vi "Calculate Joint Accelerations.vi"(0 "serial arm in":refnum<class "NI_Robotics_Serial Robot Arm.lvclass">, 5 "joint positions":dbl[](array[numeric]), 7 "joint velocities":dbl[](array[numeric]), 9 "torques":dbl[](array[numeric]), 11 "error in (no error)":errorcluster) -> (4 "serial arm out":refnum<class "NI_Robotics_Serial Robot Arm.lvclass">, 6 "joint accelerations":dbl[](array[numeric]), 15 "error out":errorcluster)   [LabVIEW 2017, in "NI_Kinematics.lvlib"]
doc: "Calculates the <B>joint accelerations</B> that result from applying <B>torques</B> to a robotic arm.\n\n<B>.m file:</B> accel"
uses:
  <vilib>/robotics/Kinematics/NI_Kinematics.lvlib
  <vilib>/robotics/Kinematics/Robot/NI_Robotics_Serial Robot Arm.lvclass
  <vilib>/Analysis/Matrix/Datatypes/RealMatrix.ctl
  <vilib>/Analysis/baseanly.llb/Real Outer Product.vi
  <vilib>/Analysis/7linalg.llb/Solve Linear Equations (single right hand).vi
  <vilib>/Analysis/baseanly.llb/Solve Linear Equations By Cholesky.vi
  <vilib>/Analysis/baseanly.llb/Real Matrix to Compact Array.vi
  <vilib>/Analysis/baseanly.llb/Real Compact Tri-Matrix Linear Eqs.vi
  <vilib>/Analysis/7linalg.llb/Solve Linear Eqs (General).vi
  <vilib>/Analysis/7linalg.llb/Solve Linear Eqs (Gen, single right hand).vi
  <vilib>/robotics/Kinematics/dyn/Inverse Dynamics (Point).vi
  <vilib>/Analysis/Matrix/Numeric/Conversions/Array To Matrix - RA2.vi
  <vilib>/robotics/Kinematics/dyn/Inverse Dynamics (Trajectory).vi
  <vilib>/Analysis/7linalg.llb/Create Special Real Matrix.vi
  <vilib>/Analysis/NI_AALBase.lvlib
  <vilib>/Analysis/Matrix/NI_Matrix.lvlib
  <vilib>/Analysis/NI_AALPro.lvlib
  <vilib>/robotics/Utilities/NI_Robotics Utilities.lvlib
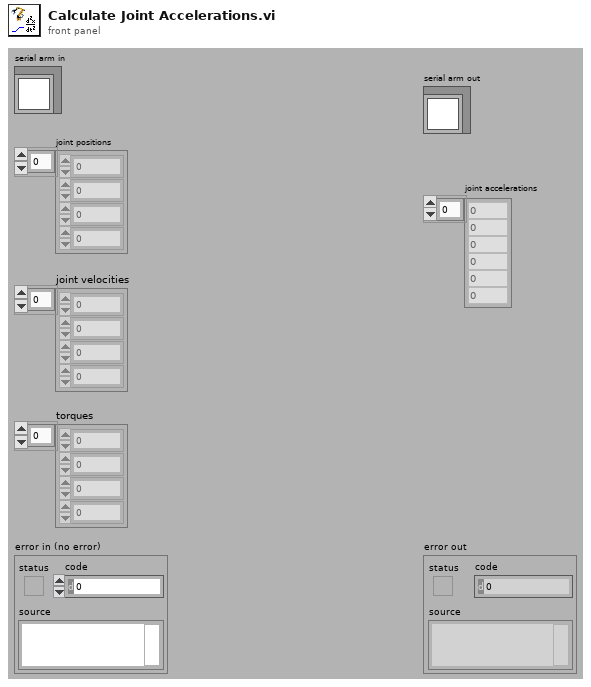
[diagram p1: front panel]
types:
  T1 = enum32{"Identity", "Diagonal", "Toepliz", "Vandermonde", "Companion"}
  T2 = typedef "NI_Matrix.lvlib/RealMatrix.ctl" = dbl[][]
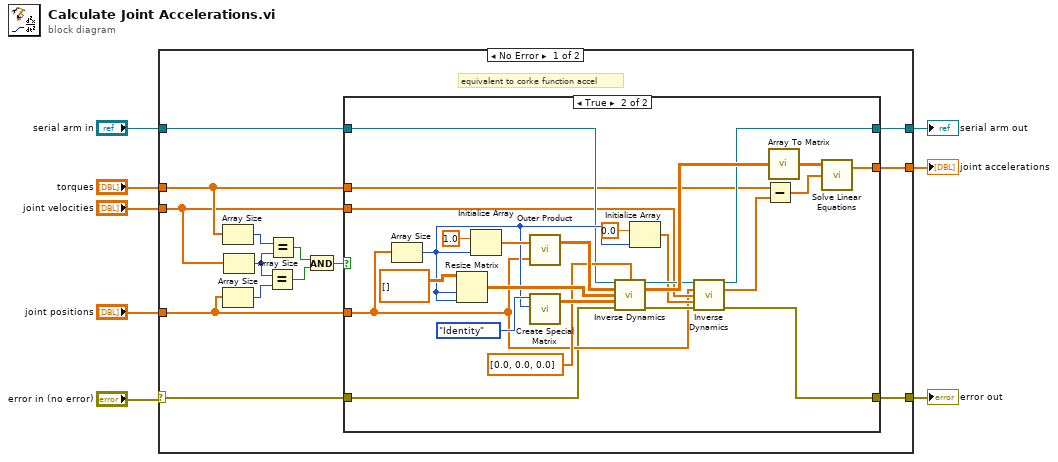
[diagram p0: block diagram]
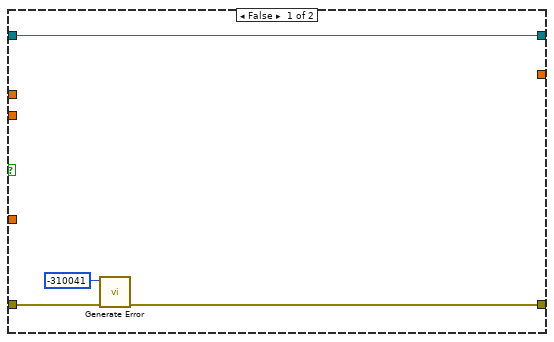
[diagram p2: hidden frame]
diagram:
  n1 = case shown="No Error" "error in (no error)" {
    selector: "error in (no error)" -> [w18 w52]
    tunnel: [w22 _] -> w8
    tunnel: "serial arm in" -> [w21 w53]
    tunnel: [w20 w53] -> w6
    tunnel: "joint positions" -> [w10 _]
    tunnel: [w19 w52] -> w5
    tunnel: "joint velocities" -> [w11 _]
    tunnel: "torques" -> [w12 _]
    frame No Error {
      # "equivalent to corke function accel"
      n2 = Array Size(array=w12) -> (size(s)=w13:i32)
      n3 = Array Size(array=w10) -> (size(s)=w14:i32)
      n4 = Array Size(array=w11) -> (size(s)=w15:i32)
      n5 = Equal?(x=w15, y=w14) -> (x = y?=w17:bool)
      n6 = Equal?(x=w13, y=w15) -> (x = y?=w16:bool)
      n7 = And(x=w16, y=w17) -> (x .and. y?=w9:bool)
      n8 = case shown="True" w9 {
        tunnel: [_ w40] -> w22
        tunnel: w21 -> [w23 w39]
        tunnel: [w23 w34] -> w20
        tunnel: [w24 w31] -> w19
        tunnel: w18 -> [w25 w27]
        tunnel: w12 -> [_ w30]
        tunnel: w11 -> [_ w29]
        tunnel: w10 -> [_ w28]
        frame False {
          n9 = call <vilib>:"Generate Error.vi"("error in (no error)"=w25, "code"=-310041) -> ("error out"=w24:errorcluster)  [unwired: 9 in]
        }
        frame True {
          n10 = Array Size(array=w28) -> (size(s)=w42:i32)
          n11 = Resize Matrix(1:w42, 2:w42, 4:T2 [] ("matrix")) -> (0:w47:T2)
          n12 = Initialize Array(1.0 ("element"), w42) -> (w50:dbl[])
          n13 = call-poly <vilib>:"Outer Product.vi"("Y Vector"=w28, "X Vector"=w50) -> ("Outer Product"=w49:T2)  [unwired: 1 out]
          n14 = call-poly <vilib>:"Create Special Matrix.vi"("matrix type"=T1."Identity", "matrix size"=w42) -> ("Special Matrix"=w45:T2)  [unwired: 3 in, 1 out]
          n15 = call-poly <vilib>:"Inverse Dynamics.vi"("serial arm in"=w39, "gravity"=dbl[] [0.0, 0.0, 0.0], "joint position trajectory"=w49, "joint velocity trajectory"=w47, "joint acceleration trajectory"=w45, "error in (no error)"=w27) -> ("serial arm out"=w35:refnum<class "NI_Robotics_Serial Robot Arm.lvclass">, "required torque trajectory"=w36:dbl[][], "error out"=w32:errorcluster)  [unwired: 7 in]
          n16 = Initialize Array(0.0 ("element"), w42) -> (w33:dbl[])
          n17 = call-poly <vilib>:"Inverse Dynamics.vi"("serial arm in"=w35, "joint positions"=w28, "joint velocities"=w29, "joint accelerations"=w33, "error in (no error)"=w32) -> ("serial arm out"=w34:refnum<class "NI_Robotics_Serial Robot Arm.lvclass">, "required torques"=w37:dbl[], "error out"=w31:errorcluster)  [unwired: 8 in]
          n18 = Subtract(x=w30, y=w37) -> (x-y=w41:dbl[])
          n19 = call-poly <vilib>:"Array To Matrix.vi"("Real 2D Array"=w36) -> ("Real Matrix"=w38:T2)
          n20 = call-poly <vilib>:"Solve Linear Equations.vi"("Known Vector"=w41, "Input Matrix"=w38) -> ("Solution Vector"=w40:dbl[])  [unwired: 1 in, 1 out]
        }
      }
    }
    frame Error {
    }
  }
  "serial arm out" <- w6
  "joint accelerations" <- w8
  "error out" <- w5
